vi "GaGe4_ConfigureTrigger.vi"(8 "error in (no error)":errorcluster, 10 "Trigger and sampling":T1={"Trig. edge"=enum."Falling", "Trig. type"=enum."Reference", "Trig. level"=2.0, "Average samples"=TRUE, "Oversample\nto match rates"=FALSE} {"Trig. level" format="%.2f"}, 11 "Handle Cluster in":T2) -> (0 "error out":errorcluster)   [LabVIEW 2015]
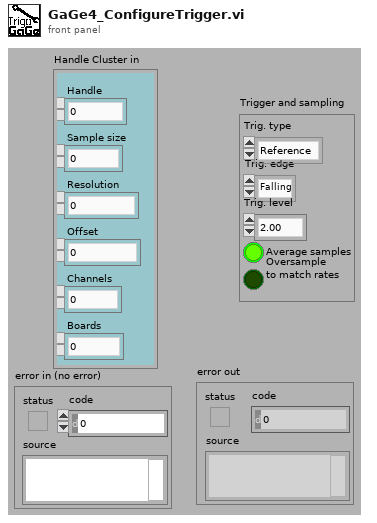
[diagram p1: front panel]
types:
  T1 = cluster{"Trig. edge":enum16{"Rising", "Falling"}, "Trig. type":enum16{"Reference", "Immediate", "Start"}, "Trig. level":sgl, "Average samples":bool, "Oversample\nto match rates":bool}
  T2 = cluster{"Handle":u32, "Sample size":u32, "Resolution":i32, "Offset":i32, "Channels":u32, "Boards":u32}
  T3 = cluster{string, i32, "Source":i32, "External Range":u32, "External Coupling":string, "External Trigger":bool, "Disable Trigger":bool}
  T4 = cluster{string, i32, "Source":i32, "External Range":u32, "External Coupling":string, "External Trigger":bool, "Disable Trigger":bool}[]
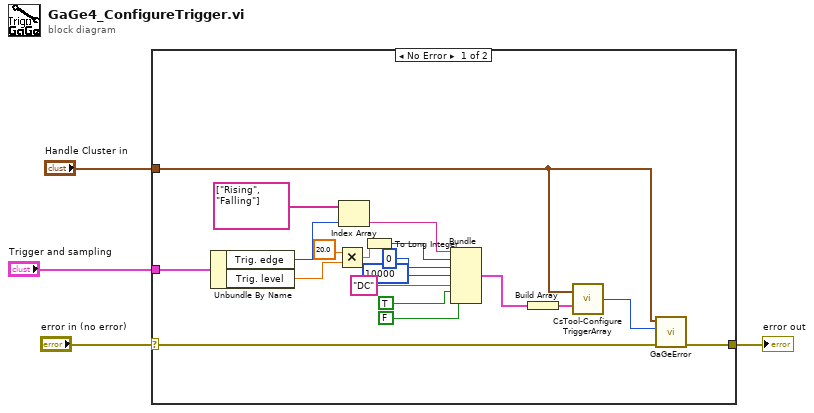
[diagram p0: block diagram]
diagram:
  n1 = case shown="No Error" "error in (no error)" {
    selector: "error in (no error)" -> [w23 w24]
    tunnel: [w22 w24] -> w3
    tunnel: "Handle Cluster in" -> [w20 _]
    tunnel: "Trigger and sampling" -> [w5 _]
    frame No Error {
      n2 = Unbundle By Name(w5) -> ("Trig. edge"=w18:enum16{"Rising", "Falling"}, "Trig. level"=w17:sgl)
      n3 = Multiply(x=sgl 20.0, y=w17) -> (x*y=w15:sgl)
      n4 = Index Array(array=string[] ["Rising", "Falling"], index=w18) -> (element=w12:string)
      n5 = To Long Integer(number=w15) -> (32bit integer=w13:i32)
      n6 = Bundle(w12, w13, "Source"=0, "External Range"=u32 10000, "External Coupling"="DC", "External Trigger"=TRUE, "Disable Trigger"=FALSE) -> (w14:T3)  [unwired: 1 out]
      n7 = Build Array(w14) -> (w9:T4)
      n8 = call "CsTool-ConfigureTriggerArray.vi"("Triggers"=w9, "Handle Cluster"=w20) -> ("Error Code"=w21:i32)
      n9 = call "GaGeError.vi"("error in (no error)"=w23, "Error Code"=w21, "Handle Cluster"=w20) -> ("error out"=w22:errorcluster)  [unwired: 3 in, 5 out]
    }
    frame Error {
    }
  }
  "error out" <- w3
